vi "WM Create Random Spectra.vi"(1 "Sampling Freq":dbl format="%.2f", 2 "Wave Spectra":dbl[](array[numeric]) format="%.2f") -> (0 "Time Series":dbl[](array[numeric]) format="%.2f")   [LabVIEW 2012]
uses:
  <vilib>/Analysis/2dsp.llb/Inverse Real FFT.vi
  <vilib>/Analysis/NI_AALPro.lvlib
  <vilib>/Analysis/NI_AALBase.lvlib
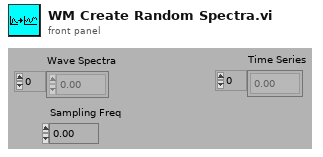
[diagram p1: front panel]
types:
  T1 = cluster{"second":i32, "minute":i32, "hour":i32, "day of month":i32, "month":i32, "year":i32, "day of week":i32, "day of year":i32, "is DST":i32}
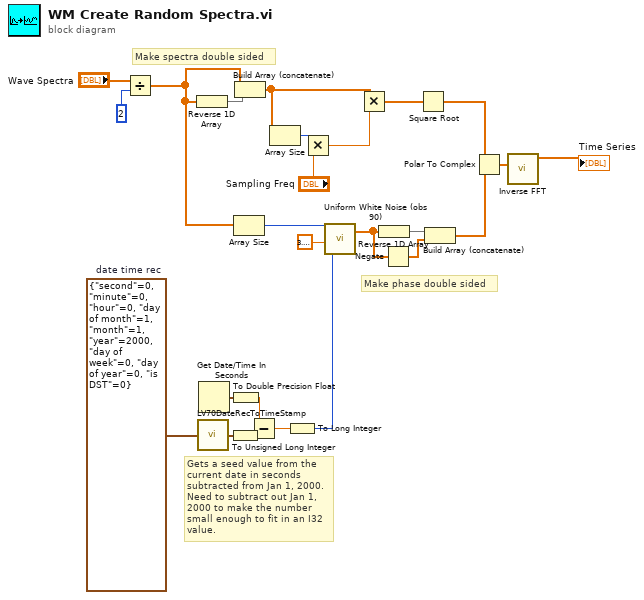
[diagram p0: block diagram]
diagram:
  w7 = T1 {"second"=0, "minute"=0, "hour"=0, "day of month"=1, "month"=1, "year"=2000, "day of week"=0, "day of year"=0, "is DST"=0}  # date time rec
  # "Gets a seed value from the current date in seconds subtracted from Jan 1, 2000.  Need to subtract out Jan 1, 2000 to make the number small enough to fit in an I32 value."
  # "Make phase double sided"
  # "Make spectra double sided"
  n1 = Divide(x="Wave Spectra", y=2) -> (x/y=w5:dbl[])
  n2 = Reverse 1D Array(array=w5) -> (reversed array=w22:dbl[])
  n3 = call <vilib>:"LV70DateRecToTimeStamp.vi"("date time rec"=w7) -> ("Time Stamp"=w2:timestamp)
  n4 = Get Date/Time In Seconds() -> (seconds since 1Jan1904=w1:timestamp)
  n5 = To Unsigned Long Integer(number=w2) -> (unsigned 32bit integer=w9:u32)
  n6 = To Double Precision Float(number=w1) -> (double precision float=w10:dbl)
  n7 = Array Size(array=w5) -> (size(s)=w12:i32)
  n8 = Build Array (concatenate)(w5, w22) -> (w13:dbl[])
  n9 = Subtract(x=w10, y=w9) -> (x-y=w8:dbl)
  n10 = Array Size(array=w13) -> (size(s)=w14:i32)
  n11 = To Long Integer(number=w8) -> (32bit integer=w6:i32)
  n12 = Multiply(x=w14, y="Sampling Freq") -> (x*y=w16:dbl)
  n13 = call <vilib>:"Uniform White Noise (obs 90).vi"("seed"=w6, "amplitude"=3.141592653589793, "samples"=w12) -> ("uniform white noise"=w19:dbl[])  [unwired: 1 out]
  n14 = Multiply(x=w13, y=w16) -> (x*y=w18:dbl[])
  n15 = Reverse 1D Array(array=w19) -> (reversed array=w21:dbl[])
  n16 = Negate(x=w19) -> (-x=w20:dbl[])
  n17 = Square Root(x=w18) -> (sqrt(x)=w11:dbl[])
  n18 = Build Array (concatenate)(w21, w20) -> (w17:dbl[])
  n19 = Polar To Complex(1:w17, 2:w11) -> (0:w23:cdb[])
  n20 = call-poly <vilib>:"Inverse FFT.vi"("FFT {X}"=w23) -> ("X"=→"Time Series":dbl[])  [unwired: 9 in, 1 out]
